vi "startTestSeries.vi"(0 "Context in":refnum<class "Context.lvclass">, 5 "Serial Number":string, 7 "Operator":string, 9 "Comments":string, 11 "error in (no error)":errorcluster) -> (4 "Context out":refnum<class "Context.lvclass">, 15 "error out":errorcluster)   [LabVIEW 2015, in "Context.lvclass"]
uses:
  Context.lvclass
  Model/Model/Model.lvclass
  State/State.lvclass
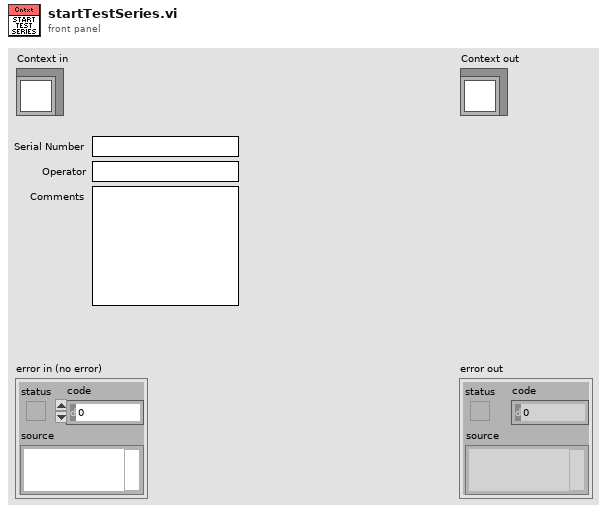
[diagram p1: front panel]
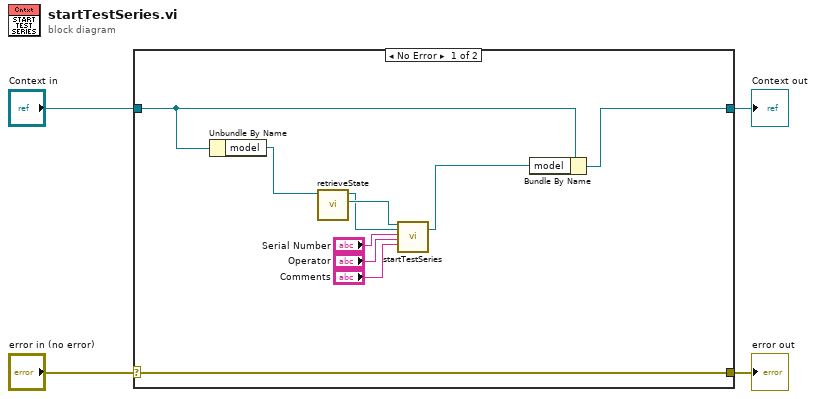
[diagram p0: block diagram]
diagram:
  n1 = case shown="No Error" "error in (no error)" {
    selector: "error in (no error)" -> [w14 w16]
    tunnel: [w14 w16] -> w3
    tunnel: [w6 w15] -> w1
    tunnel: "Context in" -> [w7 w15]
    frame No Error {
      n2 = Unbundle By Name(w7) -> ("model"=w13:refnum<class "Model.lvclass">)
      n3 = call "retrieveState.vi"("Model in"=w13) -> ("state"=w12:refnum<class "State.lvclass">, "Model out"=w11:refnum<class "Model.lvclass">)  [unwired: 8 in, 1 out]
      n4 = call-dynamic "startTestSeries.vi"("State in"=w12, "Model in"=w11, "Serial Number"="Serial Number", "Operator"="Operator", "Comments"="Comments") -> ("Model out"=w5:refnum<class "Model.lvclass">)  [unwired: 12 in, 2 out]
      n5 = Bundle By Name(cluster=w7, "model"=w5) -> (w6:refnum<class "Context.lvclass">)
    }
    frame Error {
    }
  }
  "error out" <- w3
  "Context out" <- w1
